vi "random.vi"(1 "PULSO":bool, 2 "%":dbl, 3 "in":dbl) -> (0 "out":dbl)   [LabVIEW 2018]
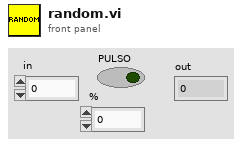
[diagram p1: front panel]
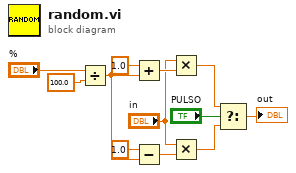
[diagram p0: block diagram]
diagram:
  n1 = Divide(x="%", y=100.0) -> (x/y=w7:dbl)
  n2 = Add(x=1.0 ("y"), y=w7) -> (x+y=w6:dbl)
  n3 = Subtract(x=1.0 ("y"), y=w7) -> (x-y=w3:dbl)
  n4 = Multiply(x="in", y=w6) -> (x*y=w5:dbl)
  n5 = Multiply(x="in", y=w3) -> (x*y=w2:dbl)
  n6 = Select(t=w5, s="PULSO", f=w2) -> (s? t:f=→"out":dbl)
